vi "Delete Query.vi"(8 "error in (no error)":errorcluster, 11 "URI in":refnum<class "URI.lvclass">) -> (0 "error out":errorcluster, 3 "URI out":refnum<class "URI.lvclass">)   [LabVIEW 2013, in "openURI.lvlib" / "URI.lvclass"]
uses:
  URI.lvclass
  components/query/URI-Component.Query.lvclass
  URI.lvclass/URI.ctl
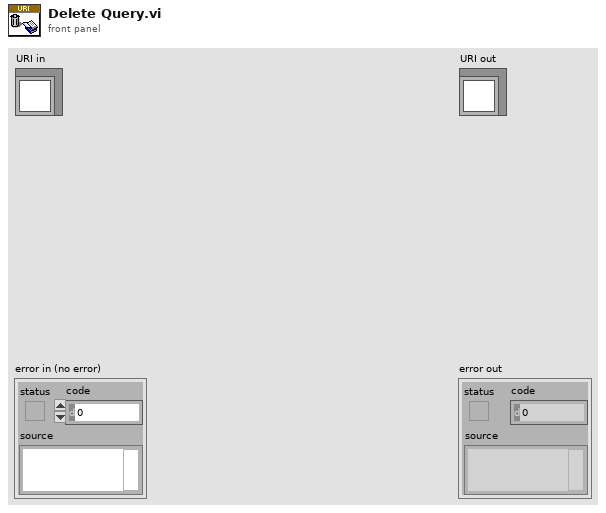
[diagram p1: front panel]
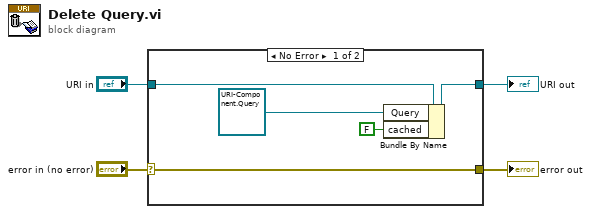
[diagram p0: block diagram]
diagram:
  n1 = case shown="No Error" "error in (no error)" {
    selector: "error in (no error)" -> [w6 w11]
    tunnel: [w6 w11] -> w3
    tunnel: [w9 w10] -> w1
    tunnel: "URI in" -> [w8 w10]
    frame No Error {
      n2 = Bundle By Name(cluster=w8, "Query"=refnum<class "URI-Component.Query.lvclass"> refnum ("openURI.lvlib:URI-Component.Query.lvclass"), "cached"=FALSE) -> (w9:refnum<class "URI.lvclass">)
    }
    frame Error {
    }
  }
  "error out" <- w3
  "URI out" <- w1
